vi "CollisionBetweenEnemyAndLine.vi"(7 "EnemyRef":refnum<class "Enemy.lvclass">, 8 "error in (no error)":errorcluster, 9 "P2":dbl[](array[numeric]), 10 "P1":dbl[](array[numeric]), 11 "Utilities in":refnum<class "Utilities.lvclass">) -> (0 "error out":errorcluster, 1 "point of collision":sgl[](array[numeric]), 2 "collision ?":bool, 3 "Utilities out":refnum<class "Utilities.lvclass">)   [LabVIEW 2020, in "Utilities.lvclass"]
uses:
  Utilities.lvclass
  Enemy_class/Enemy.lvclass
  Team_class/Team.lvclass/Team.ctl
  Object_class/Object.lvclass/Object.ctl
  Object_class/Read x.vi
  Object_class/Read y.vi
  Team_class/Read RobotRef.vi
  Robot_class/Robot.lvclass
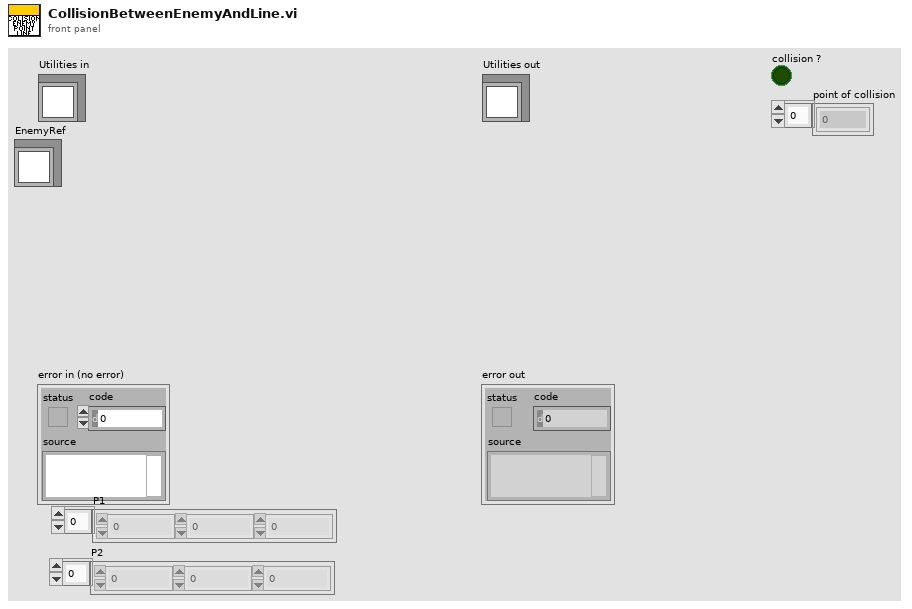
[diagram p1: front panel]
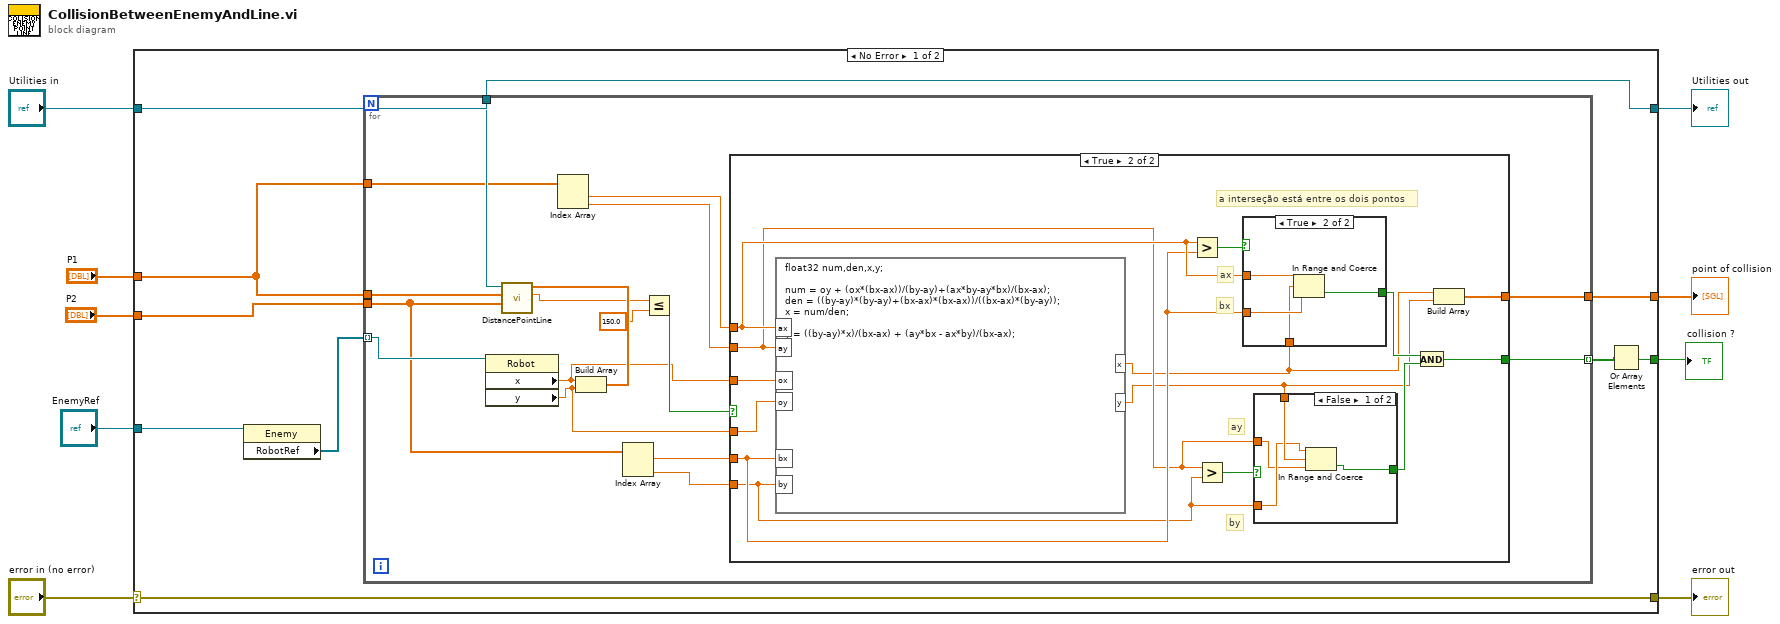
[diagram p0: block diagram]
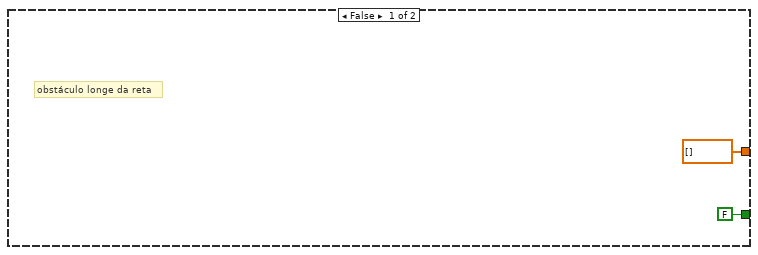
[diagram p2: hidden frame]
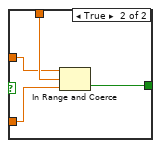
[diagram p3: hidden frame]
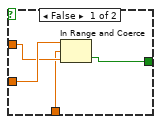
[diagram p4: hidden frame]
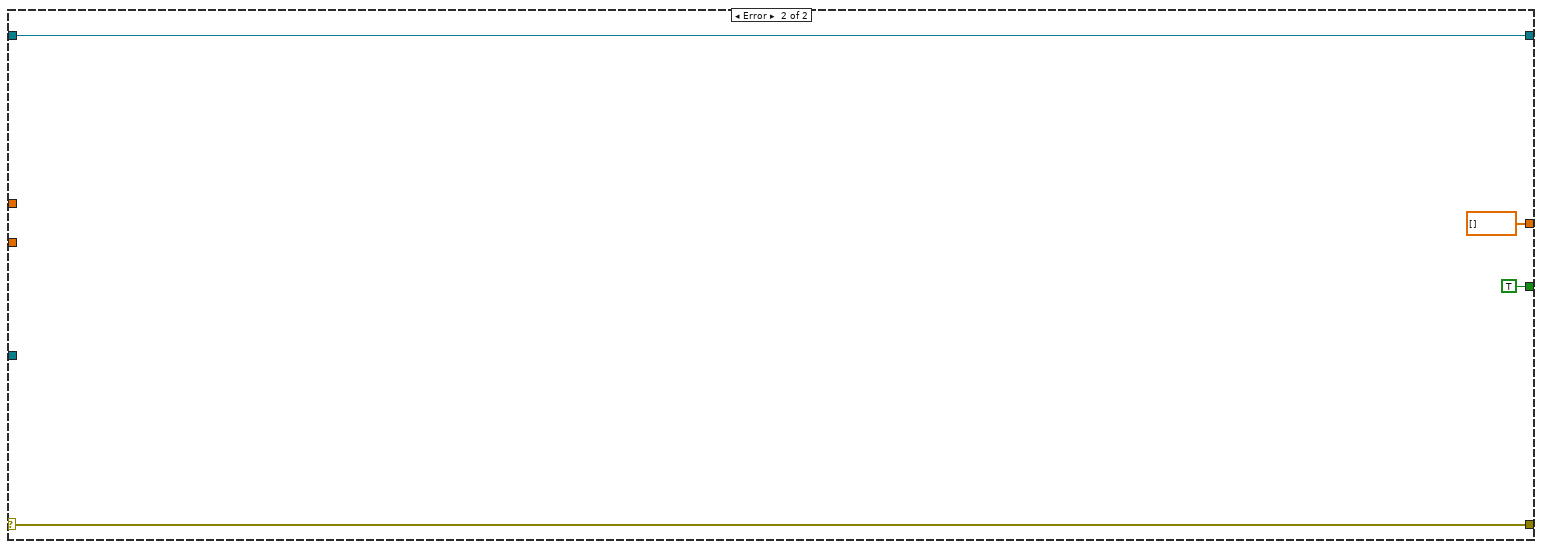
[diagram p5: hidden frame]
diagram:
  n1 = case shown="No Error" "error in (no error)" {
    selector: "error in (no error)" -> [w18 w71]
    tunnel: [w18 w71] -> w8
    tunnel: [w14 w70] -> w6
    tunnel: "Utilities in" -> [w14 w70]
    tunnel: "P2" -> [w16 _]
    tunnel: "P1" -> [w15 _]
    tunnel: [w10 TRUE] -> w3
    tunnel: [w13 sgl[] []] -> w2
    tunnel: "EnemyRef" -> [w12 _]
    frame No Error {
      n2 = property class="Enemy"(reference=w12) -> ("RobotRef"=w17:refnum<class "Robot.lvclass">[])  [unwired: 1 in, 2 out]
      n3 = for {
        tunnel: w17 -> [w33] mode=indexing
        tunnel: w15 -> [w34]
        tunnel: w16 -> [w25]
        tunnel: w14 -> [w35]
        tunnel: w15 -> [w28]
        tunnel: [w20] -> w11 mode=indexing
        tunnel: [w19] -> w13
        n4 = property class="Robot"(reference=w33) -> ("x"=w22:dbl, "y"=w21:dbl)  [unwired: 1 in, 2 out]
        n5 = Index Array(array=w28) -> (element #1=w27:dbl, element #2=w26:dbl)  [unwired: 2 in]
        n6 = Build Array(w22, w21) -> (w32:dbl[])
        n7 = call-dynamic "DistancePointLine.vi"("Q"=w32, "P2"=w25, "P1"=w34, "Utilities in"=w35) -> ("distance"=w31:dbl)  [unwired: 5 in, 2 out]
        n8 = Index Array(array=w25) -> (element #1=w24:dbl, element #2=w23:dbl)  [unwired: 2 in]
        n9 = Less Or Equal?(x=w31, y=150.0) -> (x <= y?=w29:bool)
        n10 = case shown="True" w29 {
          tunnel: w27 -> [_ w48]
          tunnel: w26 -> [_ w45]
          tunnel: w22 -> [_ w51]
          tunnel: w21 -> [_ w50]
          tunnel: w24 -> [_ w47]
          tunnel: w23 -> [_ w44]
          tunnel: [FALSE w41] -> w20
          tunnel: [sgl[] [] w38] -> w19
          frame False {
            # "obstáculo longe da reta"
          }
          frame True {
            # "a interseção está entre os dois pontos"
            # "by"
            # "ay"
            # "bx"
            # "ax"
            n11 = formula code="float32 num,den,x,y;\n\nnum = oy + (ox*(bx-ax))/(by-ay)+(ax*by-ay*bx)/(bx-ax);\nden = ((by-ay)*(by-ay)+(bx-ax)*(bx-ax))/((bx-ax)*(by-ay));\nx = num/den;\n\ny = ((by-ay)*x)/(bx-ax) + (ay*bx - ax*by)/(bx-ax);"("ax"=w48, "ay"=w45, "ox"=w51, "oy"=w50, "bx"=w47, "by"=w44) -> ("x"=w40:sgl, "y"=w39:sgl)
            n12 = Greater?(x=w48, y=w47) -> (0:w49:bool)
            n13 = Greater?(x=w45, y=w44) -> (0:w46:bool)
            n14 = case shown="True" w49 {
              tunnel: w48 -> [w62 w67]
              tunnel: w47 -> [w63 w66]
              tunnel: [w61 w65] -> w43
              tunnel: w40 -> [w60 w64]
              frame False {
                n15 = In Range and Coerce(upper limit=w63, x=w60, lower limit=w62) -> (In Range?=w61:bool)  [unwired: 1 out]
              }
              frame True {
                n16 = In Range and Coerce(upper limit=w67, x=w64, lower limit=w66) -> (In Range?=w65:bool)  [unwired: 1 out]
              }
            }
            n17 = case shown="False" w46 {
              tunnel: [w55 w59] -> w42
              tunnel: w45 -> [w52 w57]
              tunnel: w44 -> [w53 w56]
              tunnel: w39 -> [w54 w58]
              frame False {
                n18 = In Range and Coerce(upper limit=w53, x=w54, lower limit=w52) -> (In Range?=w55:bool)  [unwired: 1 out]
              }
              frame True {
                n19 = In Range and Coerce(upper limit=w57, x=w58, lower limit=w56) -> (In Range?=w59:bool)  [unwired: 1 out]
              }
            }
            n20 = And(x=w43, y=w42) -> (x .and. y?=w41:bool)
            n21 = Build Array(w40, w39) -> (w38:sgl[])
          }
        }
      }
      n22 = Or Array Elements(Boolean array=w11) -> (logical OR=w10:bool)
    }
    frame Error {
    }
  }
  "error out" <- w8
  "Utilities out" <- w6
  "collision ?" <- w3
  "point of collision" <- w2
